vi "BuildCall.vi"(7 "PythonConverter_BD in":refnum<class "PyConvBD.lvclass">, 8 "error in":errorcluster, 11 "SubVI in":refnum<class "SubVI.lvclass">) -> (0 "error out":errorcluster, 3 "SubVI out":refnum<class "SubVI.lvclass">, 5 "PythonConverter_BD out":refnum<class "PyConvBD.lvclass">)   [LabVIEW 2014, in "Raspberry Pi Compatible Compiler for LabVIEW.lvlib" / "SubVI.lvclass"]
uses:
  SubVI.lvclass
  Python/PythonConverter_BD/PyConvBD.lvclass
  SubVI.lvclass/SubVI.ctl
  Python/PythonConverter_BD/TypeDefs/NodeCall_TD.ctl
  Python/Parsing/ListTypesTD.ctl
  Node/Node.lvclass
  Raspberry Pi Compatible Compiler for LabVIEW.lvlib
  Python/Parsing/Python Functions.lvlib
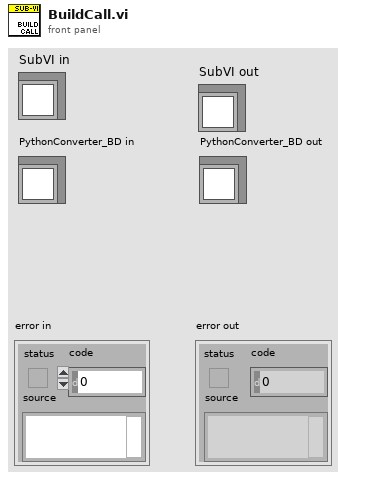
[diagram p1: front panel]
types:
  T1 = typedef "Raspberry Pi Compatible Compiler for LabVIEW.lvlib/Python Functions.lvlib/ListTypesTD.ctl" = enum16{"list", "tuple", "parameter list", "output list", "return values"}
  T2 = typedef "Raspberry Pi Compatible Compiler for LabVIEW.lvlib/NodeCall_TD.ctl" = cluster{"call":string, "collect":string, "Threaded":bool, "branches":string[]}
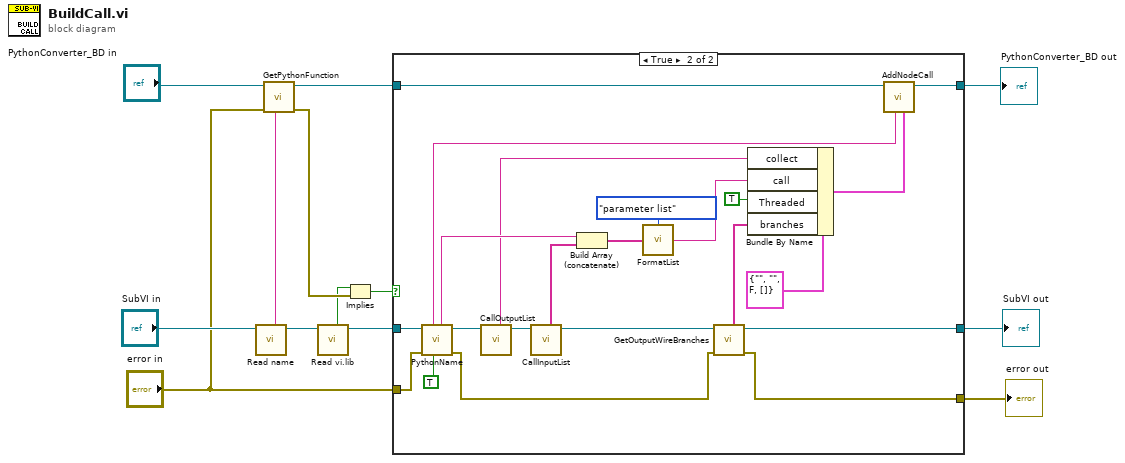
[diagram p0: block diagram]
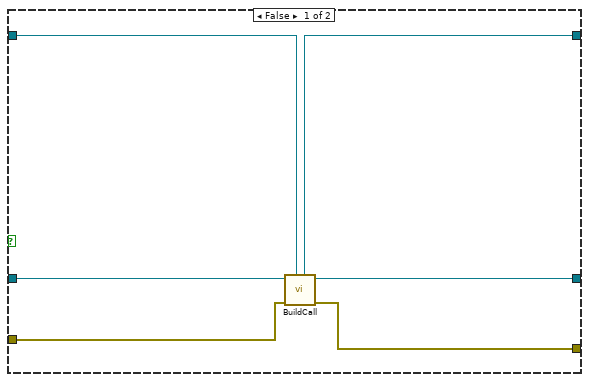
[diagram p2: hidden frame]
diagram:
  n1 = call-dynamic "Read name.vi"("SubVI in"="SubVI in") -> ("SubVI out"=w12:refnum<class "SubVI.lvclass">, "name"=w10:string)  [unwired: 7 in]
  n2 = call "GetPythonFunction.vi"("function name"=w10, "error in"="error in", "PythonConverter_BD in"="PythonConverter_BD in") -> ("error out"=w13:errorcluster, "PythonConverter_BD out"=w4:refnum<class "PyConvBD.lvclass">)  [unwired: 4 in, 1 out]
  n3 = call "Read vi.lib.vi"("SubVI in"=w12) -> ("SubVI out"=w7:refnum<class "SubVI.lvclass">, "vi.lib"=w11:bool)  [unwired: 7 in]
  n4 = Implies(1:w13, 2:w11) -> (0:w6:bool)
  n5 = case shown="True" w6 {
    tunnel: [w16 w28] -> w1
    tunnel: w7 -> [w19 w41]
    tunnel: [w18 w30] -> w2
    tunnel: "error in" -> [w17 w24]
    tunnel: w4 -> [w14 w23]
    tunnel: [w15 w20] -> w3
    frame False {
      n6 = call-parent "BuildCall.vi"("PythonConverter_BD in"=w14, "error in"=w17, "Node in"=w19) -> ("error out"=w16:errorcluster, "Node out"=w18:refnum<class "SubVI.lvclass">, "PythonConverter_BD out"=w15:refnum<class "PyConvBD.lvclass">)  [unwired: 6 in]
    }
    frame True {
      n7 = call-dynamic "PythonName.vi"("add self"=TRUE, "error in"=w24, "Node in"=w41) -> ("error out"=w29:errorcluster, "Node out"=w26:refnum<class "SubVI.lvclass">, "name"=w40:string, "UID"=w22:string)  [unwired: 5 in]
      n8 = call-dynamic "CallOutputList.vi"("SubVI in"=w26) -> ("SubVI out"=w25:refnum<class "SubVI.lvclass">, "call outputs"=w33:string)  [unwired: 7 in]
      n9 = call-dynamic "CallInputList.vi"("SubVI in"=w25) -> ("SubVI out"=w31:refnum<class "SubVI.lvclass">, "call inputs"=w39:string[])  [unwired: 7 in]
      n10 = Build Array (concatenate)(w40, w39) -> (w34:string[])
      n11 = call "FormatList.vi"("values"=w34, "type"=ListTypesTD."parameter list") -> ("python object"=w32:string)
      n12 = call-dynamic "GetOutputWireBranches.vi"("error in"=w29, "Node in"=w31) -> ("error out"=w28:errorcluster, "Node out"=w30:refnum<class "SubVI.lvclass">, "branches"=w27:string[])  [unwired: 5 in]
      n13 = Bundle By Name(cluster=T2 {"call"="", "collect"="", "Threaded"=FALSE, "branches"=[]} ("call"), "collect"=w33, "call"=w32, "Threaded"=TRUE, "branches"=w27) -> (w21:T2)
      n14 = call "AddNodeCall.vi"("call"=w21, "name"=w22, "PythonConverter_BD in"=w23) -> ("PythonConverter_BD out"=w20:refnum<class "PyConvBD.lvclass">)  [unwired: 5 in, 1 out]
    }
  }
  "error out" <- w1
  "SubVI out" <- w2
  "PythonConverter_BD out" <- w3
